vi "modify channel test.vi"() -> ()   [LabVIEW 2013, in "Tag Bus Web Interface tests.lvlib"]
uses:
  Tag Bus Web Interface tests.lvlib
  <vilib>/NI/Tag Bus Module Framework/channel/channel classification.ctl
  configuration/Tag Bus Web Interface configuration.lvclass
  configuration/Tag Bus Web Interface configuration.lvclass/Tag Bus Web Interface configuration.ctl
  <vilib>/NI/Tag Bus Module Framework/channel/TBM channel.lvclass/TBM channel.ctl
  <vilib>/NI/Tag Bus/tag/tag descriptor.lvclass/tag descriptor.ctl
  <vilib>/NI/Tag Bus Module Framework/channel/Read channel classification.vi
  <vilib>/NI/Tag Bus Module Framework/channel/Write channel classification.vi
  <vilib>/NI/Tag Bus/tag/read tag name.vi
  configuration/Write channels.vi
  <vilib>/NI/Tag Bus Module Framework/channel/TBM channel.lvclass
  <vilib>/NI/Configuration Framework/serializable configuration/NISE_CEF_serializable configuration.lvclass
panel:
  out "rename success":bool
  out "no err":errorcluster
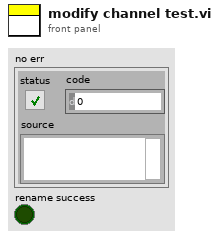
[diagram p1: front panel]
types:
  T1 = typedef "TBM channel.lvclass/channel classification.ctl" = enum16{"input data", "output data", "processing parameter", "processing result"}
  T2 = typedef "tag bus.lvlib/tag descriptor.lvclass/Data Type.ctl" = enum16{"Double", "Single", "I64", "I32", "I16", "I8", "U64", "U32", "U16", "U8", "Boolean", "String", "Array of Double", "Array of Single", "Array of I64", "Array of I32", "Array of I16", "Array of I8", "Array of U64", "Array of U32", "Array of U16", "Array of U8", "Array of Boolean", "Array of String"}
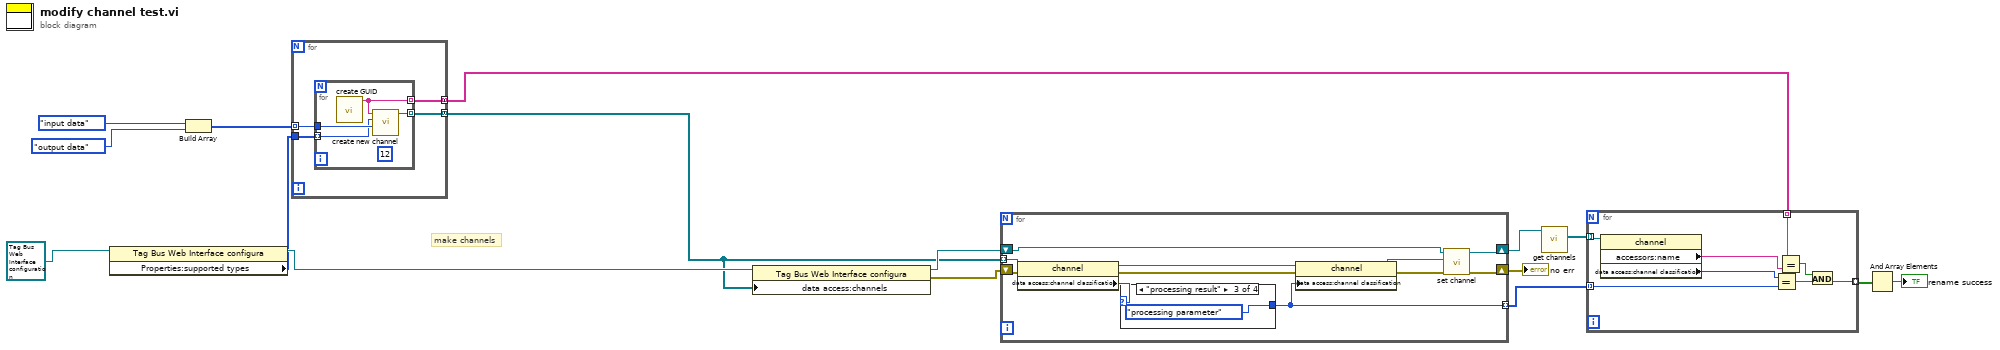
[diagram p0: block diagram]
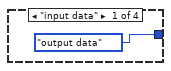
[diagram p2: hidden frame]
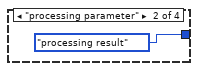
[diagram p3: hidden frame]
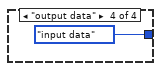
[diagram p4: hidden frame]
diagram:
  # "make channels"
  n1 = property class="Tag Bus Web Interface configura"(reference=refnum<class "Tag Bus Web Interface configuration.lvclass"> refnum ("tag bus configurable plugin module configuration")) -> (reference out=w13:refnum<class "Tag Bus Web Interface configuration.lvclass">, "Properties:supported types"=w12:T2[])  [unwired: 1 in, 1 out]
  n2 = Build Array(channel_classification."input data" ("channel classification"), channel_classification."output data" ("channel classification")) -> (w14:T1[])
  n3 = for {
    tunnel: w14 -> [w20] mode=indexing
    tunnel: [w18] -> w1 mode=concatenating
    tunnel: w12 -> [w19]
    tunnel: [w17] -> w5 mode=concatenating
    n4 = for {
      tunnel: w20 -> [w23]
      tunnel: [w24] -> w18 mode=indexing
      tunnel: w19 -> [w22] mode=indexing
      tunnel: [w21] -> w17 mode=indexing
      (unwired) 12
      n5 = call <vilib>:"create GUID.vi"() -> ("uuid"=w21:string)  [unwired: 11 in]
      n6 = call <vilib>:"create new channel.vi"("channel classification"=w23, "data type"=w22, "channel name"=w21) -> ("channel"=w24:refnum<class "TBM channel.lvclass">)  [unwired: 8 in]
    }
  }
  n7 = property class="Tag Bus Web Interface configura"(reference=w13, "data access:channels"=w1) -> (reference out=w2:refnum<class "Tag Bus Web Interface configuration.lvclass">, error out=w3:errorcluster)  [unwired: 1 in]
  n8 = for {
    shift-right: [w34] -> w11
    shift-left: w2 -> [w35]
    shift-right: [w33] -> w10
    shift-left: w3 -> [w32]
    tunnel: w1 -> [w30] mode=indexing
    tunnel: [w25] -> w6 mode=indexing
    n9 = property class="channel"(reference=w30, error in=w32) -> (reference out=w28:refnum<class "TBM channel.lvclass">, error out=w31:errorcluster, "data access:channel classification"=w26:T1)
    n10 = case shown="\"processing result\"" w26 {
      tunnel: [channel_classification."output data" ("channel classification") channel_classification."processing result" ("channel classification") channel_classification."processing parameter" ("channel classification") channel_classification."input data" ("channel classification")] -> w25
      frame "input data" {
      }
      frame "processing parameter" {
      }
      frame "processing result" {
      }
      frame "output data" {
      }
    }
    n11 = property class="channel"(reference=w28, error in=w31, "data access:channel classification"=w25) -> (reference out=w27:refnum<class "TBM channel.lvclass">, error out=w29:errorcluster)
    n12 = call "set channel.vi"("error in"=w29, "TBM channel in"=w27, "Tag Bus Web Interface configuration in"=w35) -> ("error out"=w33:errorcluster, "Tag Bus Web Interface configuration out"=w34:refnum<class "Tag Bus Web Interface configuration.lvclass">)  [unwired: 7 in]
  }
  "no err" <- w10
  n13 = call-dynamic "get channels.vi"("Tag Bus Web Interface configuration in"=w11) -> ("channels"=w9:refnum<class "TBM channel.lvclass">[])  [unwired: 9 in, 1 out]
  n14 = for {
    tunnel: w9 -> [w46] mode=indexing
    tunnel: [w45] -> w8 mode=indexing
    tunnel: w6 -> [w44] mode=indexing
    tunnel: w5 -> [w41] mode=indexing
    n15 = property class="channel"(reference=w46) -> ("accessors:name"=w42:string, "data access:channel classification"=w43:T1)  [unwired: 1 in, 2 out]
    n16 = Equal?(x=w43, y=w44) -> (x = y?=w47:bool)
    n17 = Equal?(x=w41, y=w42) -> (x = y?=w40:bool)
    n18 = And(x=w40, y=w47) -> (x .and. y?=w45:bool)
  }
  n19 = And Array Elements(Boolean array=w8) -> (logical AND=→"rename success":bool)
